vi "SetTrigger.vi"(8 "error in":errorcluster, 10 "trig":T1={"trigger"=TRUE, "Delay (us)"=0.0, "Out 1"=enum."Imaging", "Out 2"=enum."Imaging"}, 11 "camera.nit in":refnum<class "camera.lvclass">) -> (0 "error out":errorcluster)   [LabVIEW 2020, in "camera.lvclass"]
uses:
  camera.lvclass
  _controls/trigger.ctl
  _controls/trigger.mode.ctl
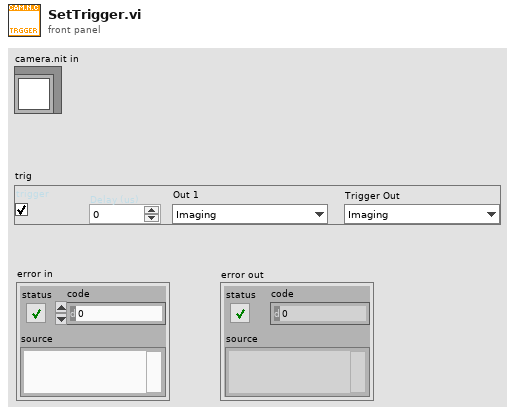
[diagram p1: front panel]
types:
  T1 = typedef "trigger.ctl" = cluster{"trigger":bool, "Delay (us)":dbl, "Out 1":T2, "Out 2":T2}
  T2 = typedef "trigger.mode.ctl" = enum16{"Exposition", "Readout", "Imaging", "Trigger Ready", "Mirror Trigger Input", "Output High"}
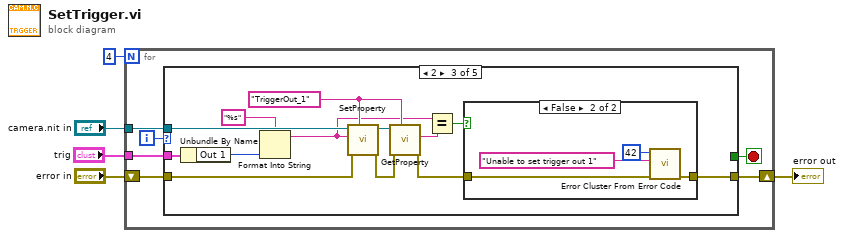
[diagram p0: block diagram]
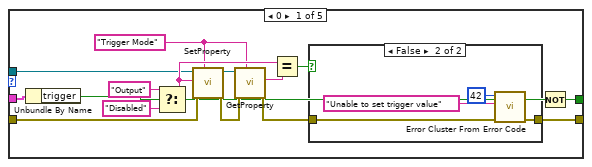
[diagram p2: hidden frame]
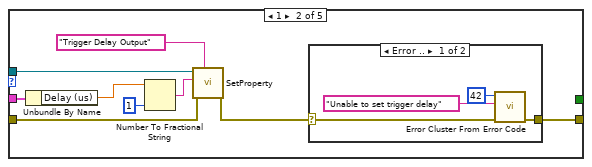
[diagram p4: hidden frame]
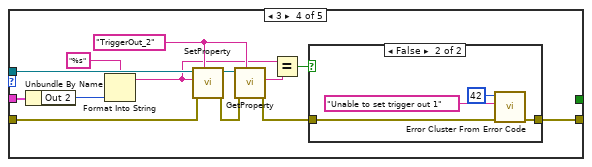
[diagram p7: hidden frame]
diagram:
  n1 = for {
    N: 4 -> [_]
    tunnel: "trig" -> [w11]
    tunnel: "camera.nit in" -> [w9]
    shift-right: [w10] -> w5
    shift-left: "error in" -> [w8]
    i -> [w7]
    stop <- w6 stop-if-true
    n2 = case shown="2" w7 {
      tunnel: w11 -> [w20 w39 w56 w73 _]
      tunnel: [w19 w38 w55 w72 w79] -> w10
      tunnel: w9 -> [w16 w36 w54 w71 _]
      tunnel: w8 -> [w14 w35 w53 w70 w79]
      tunnel: [w12 _ _ _ _] -> w6
      frame 0 {
        w17 = "Trigger Mode" ("pPrp")
        n3 = Unbundle By Name(w20) -> ("trigger"=w13:bool)
        n4 = Select(t="Output" ("Value"), s=w13, f="Disabled") -> (s? t:f=w23:string)
        n5 = call-dynamic "SetProperty.vi"("Property"=w17, "error in"=w14, "Value"=w23, "camera.nit in"=w16) -> ("error out"=w15:errorcluster)  [unwired: 7 in]
        n6 = call-dynamic "GetProperty.vi"("Property"=w17, "error in"=w15, "camera.nit in"=w16) -> ("error out"=w18:errorcluster, "value"=w24:string)  [unwired: 7 in]
        n7 = Equal?(x=w23, y=w24) -> (x = y?=w25:bool)
        n8 = case shown="False" w25 {
          tunnel: w18 -> [w26 w30]
          tunnel: [w26 w28] -> w19
          frame True {
          }
          frame False {
            n9 = call <vilib>:"Error Cluster From Error Code.vi"("error in (no error)"=w30, "error message (\"\")"="Unable to set trigger value" ("error message (\"\")"), "error code (0)"=42) -> ("error out"=w28:errorcluster)  [unwired: 6 in]
          }
        }
        n10 = Not(x=w13) -> (.not. x?=w12:bool)
      }
      frame 1 {
        n11 = Unbundle By Name(w39) -> ("Delay (us)"=w34:dbl)
        n12 = Number To Fractional String(number=w34, precision (6)=i16 1) -> (F-format string=w33:string)  [unwired: 2 in]
        n13 = call-dynamic "SetProperty.vi"("Property"="Trigger Delay Output" ("pPrp"), "error in"=w35, "Value"=w33, "camera.nit in"=w36) -> ("error out"=w31:errorcluster)  [unwired: 7 in]
        n14 = case shown="Error .." w31 {
          selector: w31 -> [w40 w44]
          tunnel: [w42 w44] -> w38
          frame Error {
            n15 = call <vilib>:"Error Cluster From Error Code.vi"("error in (no error)"=w40, "error message (\"\")"="Unable to set trigger delay" ("error message (\"\")"), "error code (0)"=42) -> ("error out"=w42:errorcluster)  [unwired: 6 in]
          }
          frame No Error {
          }
        }
      }
      frame 2 {
        w49 = "TriggerOut_1" ("pPrp")
        n16 = Unbundle By Name(w56) -> ("Out 1"=w47:T2)
        n17 = Format Into String(format string="%s", w47) -> (resulting string=w45:string)  [unwired: 2 in, 1 out]
        n18 = call-dynamic "SetProperty.vi"("Property"=w49, "error in"=w53, "Value"=w45, "camera.nit in"=w54) -> ("error out"=w48:errorcluster)  [unwired: 7 in]
        n19 = call-dynamic "GetProperty.vi"("Property"=w49, "error in"=w48, "camera.nit in"=w54) -> ("error out"=w50:errorcluster, "value"=w51:string)  [unwired: 7 in]
        n20 = Equal?(x=w45, y=w51) -> (x = y?=w52:bool)
        n21 = case shown="False" w52 {
          tunnel: w50 -> [w57 w61]
          tunnel: [w57 w59] -> w55
          frame True {
          }
          frame False {
            n22 = call <vilib>:"Error Cluster From Error Code.vi"("error in (no error)"=w61, "error message (\"\")"="Unable to set trigger out 1" ("error message (\"\")"), "error code (0)"=42) -> ("error out"=w59:errorcluster)  [unwired: 6 in]
          }
        }
      }
      frame 3 {
        w66 = "TriggerOut_2" ("pPrp")
        n23 = Unbundle By Name(w73) -> ("Out 2"=w64:T2)
        n24 = Format Into String(format string="%s", w64) -> (resulting string=w62:string)  [unwired: 2 in, 1 out]
        n25 = call-dynamic "SetProperty.vi"("Property"=w66, "error in"=w70, "Value"=w62, "camera.nit in"=w71) -> ("error out"=w65:errorcluster)  [unwired: 7 in]
        n26 = call-dynamic "GetProperty.vi"("Property"=w66, "error in"=w65, "camera.nit in"=w71) -> ("error out"=w67:errorcluster, "value"=w68:string)  [unwired: 7 in]
        n27 = Equal?(x=w62, y=w68) -> (x = y?=w69:bool)
        n28 = case shown="False" w69 {
          tunnel: w67 -> [w74 w78]
          tunnel: [w74 w76] -> w72
          frame True {
          }
          frame False {
            n29 = call <vilib>:"Error Cluster From Error Code.vi"("error in (no error)"=w78, "error message (\"\")"="Unable to set trigger out 1" ("error message (\"\")"), "error code (0)"=42) -> ("error out"=w76:errorcluster)  [unwired: 6 in]
          }
        }
      }
      frame Default {
      }
    }
  }
  "error out" <- w5
